vi "Shutdown.vi"(8 "error in (no error)":errorcluster, 11 "ConsoleInterface in":refnum<class "ConsoleSession.lvclass">) -> (0 "error out":errorcluster)   [LabVIEW 2020, in "MVA Framework.lvlib" / "ConsoleView.lvlib" / "ConsoleSession.lvclass"]
doc: "Shutdown the view and associated sink. Calling this method is not required - the view and associated sink will be closed on shutdown of the owning logger. The method is provided for a use case where the view and sink should be closed before the logger."
uses:
  ConsoleSession.lvclass
  ConsoleSession.lvclass/ConsoleSession.ctl
  Composed Log/Types/MessageCluster.ctl
  Composed Log/Composed Log.lvlib
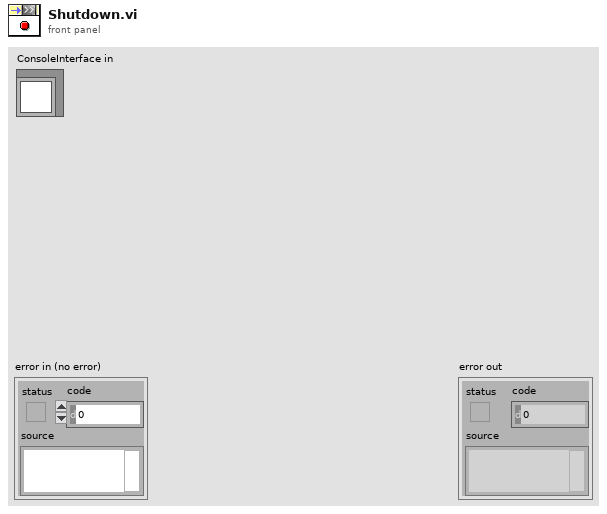
[diagram p1: front panel]
types:
  T1 = typedef "MVA Framework.lvlib/Composed Log.lvlib/MessageCluster.ctl" = cluster{"Message":string, "Data":variant}
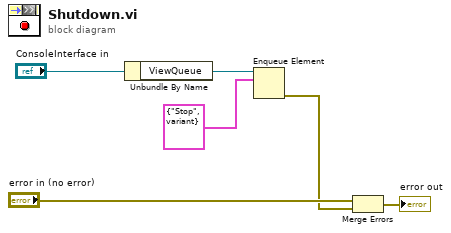
[diagram p0: block diagram]
diagram:
  n1 = Unbundle By Name("ConsoleInterface in") -> ("ViewQueue"=w4:refnum<queue>)
  n2 = Enqueue Element(queue=w4, element=T1 {"Message"="Stop", "Data"=variant}) -> (error out=w1:errorcluster)  [unwired: 2 in, 2 out]
  n3 = Merge Errors("error in (no error)", w1) -> (→"error out":errorcluster)
